vi "Set_Pulse_Manual.vi"() -> ()   [LabVIEW 2021]
uses:
  Drivers/Arduino_Pulse_Generator/Configurate/Channel_Pulse_Stream.ctl
  acefff95-97c1-4a03-be14-0b511ca0e7e1.vi
  db7f351c-eeeb-4ffc-aff2-0ba6d56ef54f.vi
  <vilib>/Comparison/Less/Less Functor/Less Functor.lvclass
panel:
  in  "Filename (.ini)":string="Config_Ver_1\\pulse_sequence.ini"
  out "Initial Array":T1[](array[typedef]) {"channel" min=2 max=13 step=1}
  in  "Reset All":bool
  in  "Reset Channel":bool
  out "Type of channel":string[](array[string])
  out "Times vs channel":dbl[][](array[numeric])
  in  "End configuration":bool
  in  "Stop":dbl
  in  "Start":dbl
  in  "Add Step":bool
  in  "Add Pulse":bool
  in  "Type of channel":u8(ring) items=["probe"=4, "pump"=6, "x pulse"=7]
  # "Note that units of time are not specified there.\nRemember that minimal pulse length is about 3,8 us."
  # "Add pulse with specific type\nbegining (start) and end (stop)"
  # "Add step with specific type\nand time (start)"
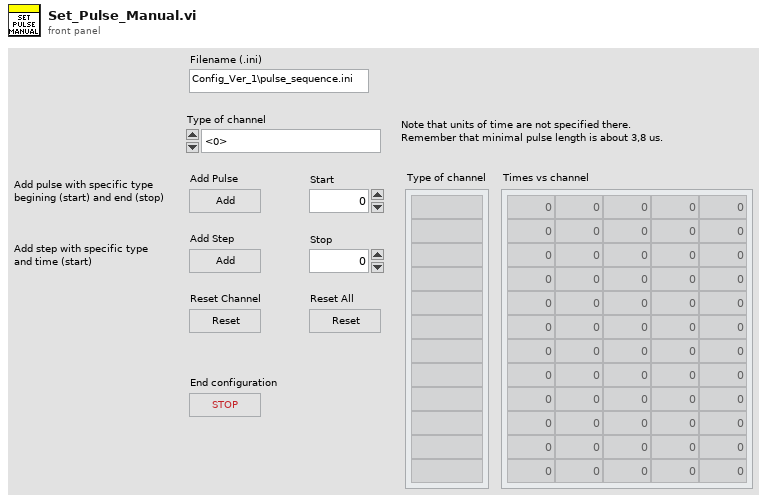
[diagram p1: front panel]
types:
  T1 = typedef "Channel_Pulse_Stream.ctl" = cluster{"Times":dbl[], "channel":u8}
  T2 = typedef "Channels_Map.ctl" = T3[]
  T3 = typedef "Channel_Cluster.ctl" = cluster{"Channel name":string, "Channel":u8}
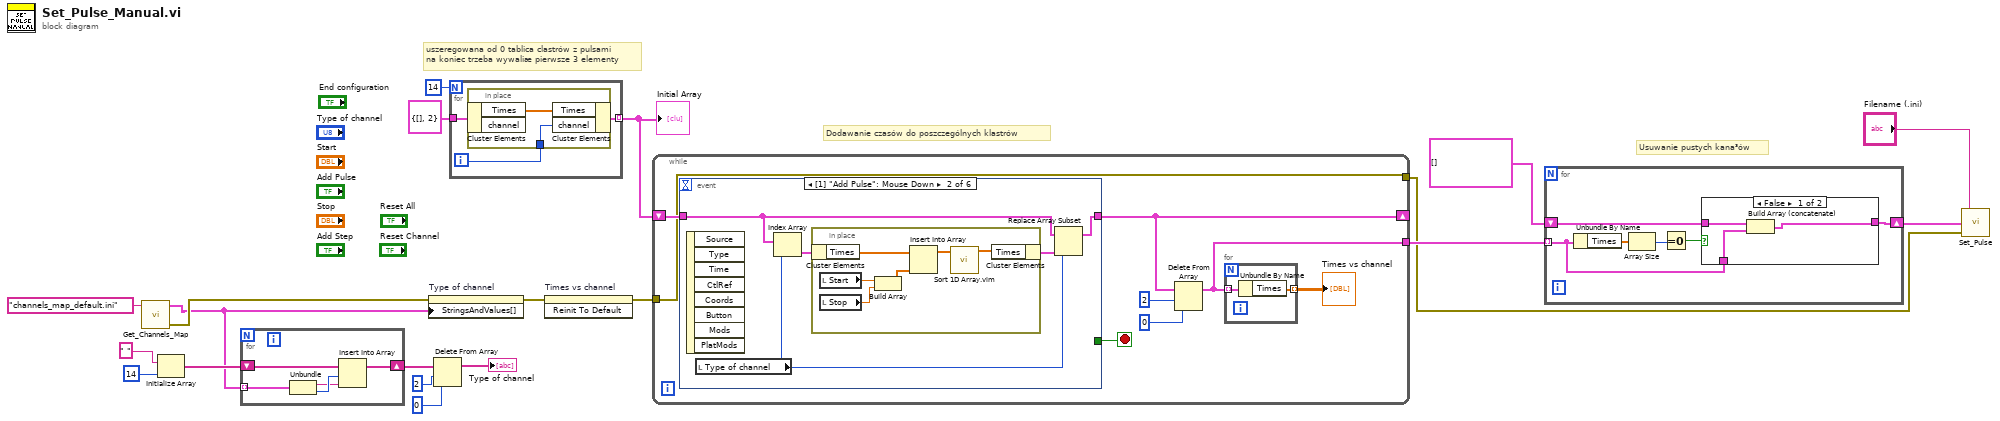
[diagram p0: block diagram]
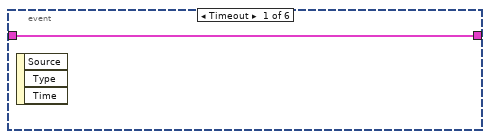
[diagram p3: hidden frame]
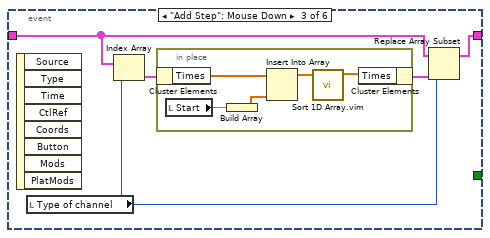
[diagram p4: hidden frame]
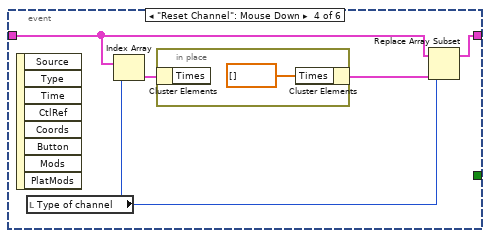
[diagram p5: hidden frame]
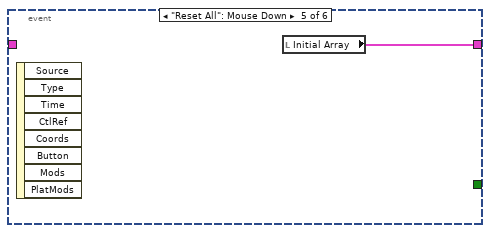
[diagram p6: hidden frame]
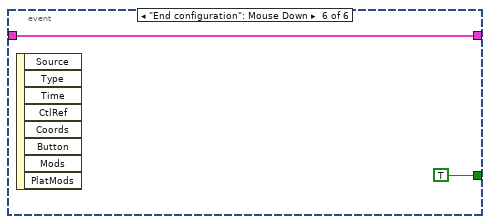
[diagram p7: hidden frame]
diagram:
  # "Usuwanie pustych kana³ów"
  # "uszeregowana od 0 tablica clastrów z pulsami\nna koniec trzeba wywaliæ pierwsze 3 elementy"
  # "Dodawanie czasów do poszczególnych klastrów"
  n1 = call "Get_Channels_Map.vi"("Filename (.ini)"="channels_map_default.ini") -> ("error out"=w6:errorcluster, "Channels Map"=w5:T2)  [unwired: 3 in]
  n2 = Initialize Array(" ", 14 ("dimension size")) -> (w13:string[])
  n3 = for {
    tunnel: w5 -> [w23] mode=indexing
    shift-right: [w22] -> w12
    shift-left: w13 -> [w25]
    n4 = Unbundle(w23) -> ("Channel name"=w21:string, "Channel"=w24:u8)
    n5 = Insert Into Array(array=w25, index=w24, new element=w21) -> (w22:string[])
  }
  n6 = property on="Type of channel" class="Ring (strict)"(error in=w6, "StringsAndValues[]"=w5) -> (error out=w17:errorcluster)  [unwired: 1 in, 1 out]
  n7 = Delete From Array(array=w12, length=2, index=0) -> (array with subset deleted=→"Type of channel":string[])  [unwired: 1 out]
  n8 = for {
    N: 14 -> [_]
    tunnel: T1 {"Times"=[], "channel"=2} ("Channel pulse stream") -> [w28]
    tunnel: [w27] -> w18 mode=indexing
    i -> [w26]
    n9 = in-place {
      in-place-border: w26 -> [w30]
      n10 = in-place-cluster #1(w28) -> ("Times"=w29:dbl[])  [unwired: 1 out]
      n11 = in-place-cluster #1("Times"=w29, "channel"=w30) -> (w27:T1)
    }
  }
  "Initial Array" <- w18
  n12 = invoke on="Times vs channel" class="Arr (strict)" method="Reinit To Default"(error in=w17) -> (error out=w16:errorcluster)  [unwired: 2 in, 2 out]
  n13 = while {
    shift-right: [w34] -> _
    shift-left: w18 -> [w38]
    tunnel: [w32] -> w8
    tunnel: w16 -> [w31]
    tunnel: [w31] -> w2
    stop <- w37 stop-if-true
    n14 = event shown="[1] \"Add Pulse\": Mouse Down" {
      selector: _ -> [_ _ _ _ _ _]
      dyn-events: _ -> [_ _ _ _ _ _]
      timeout: _ -> [_ _ _ _ _ _]
      tunnel: w38 -> [w41 w44 w55 w65 _ w71]
      tunnel: [w41 w42 w53 w63 w69 w71] -> w34
      tunnel: [_ _ _ _ _ TRUE] -> w37
      event Timeout {
        n15 = event-data() -> ()  [unwired: 1 in, 3 out]
      }
      event "Add Pulse": Mouse Down {
        n16 = event-data() -> ()  [unwired: 1 in, 8 out]
        n17 = local read "Type of channel"() -> (w43:u8)
        n18 = Index Array(array=w44, index=w43) -> (element=w46:T1)
        n19 = in-place {
          n20 = in-place-cluster #2(w46) -> ("Times"=w50:dbl[])
          n21 = local read "Start"() -> (w51:dbl)
          n22 = local read "Stop"() -> (w52:dbl)
          n23 = Build Array(w51, w52) -> (w49:dbl[])
          n24 = Insert Into Array(array=w50, new element=w49) -> (w48:dbl[])  [unwired: 1 in]
          n25 = call "Sort 1D Array.vim"("unsorted array"=w48) -> ("sorted array"=w47:dbl[])  [unwired: 10 in]
          n26 = in-place-cluster #2("Times"=w47) -> (w45:T1)
        }
        n27 = Replace Array Subset(array=w44, new element=w45, index=w43) -> (w42:T1[])
      }
      event "Add Step": Mouse Down {
        n28 = event-data() -> ()  [unwired: 1 in, 8 out]
        n29 = local read "Type of channel"() -> (w54:u8)
        n30 = Index Array(array=w55, index=w54) -> (element=w57:T1)
        n31 = in-place {
          n32 = in-place-cluster #3(w57) -> ("Times"=w61:dbl[])
          n33 = local read "Start"() -> (w62:dbl)
          n34 = Build Array(w62) -> (w60:dbl[])
          n35 = Insert Into Array(array=w61, new element=w60) -> (w59:dbl[])  [unwired: 1 in]
          n36 = call "Sort 1D Array.vim"("unsorted array"=w59) -> ("sorted array"=w58:dbl[])  [unwired: 10 in]
          n37 = in-place-cluster #3("Times"=w58) -> (w56:T1)
        }
        n38 = Replace Array Subset(array=w55, new element=w56, index=w54) -> (w53:T1[])
      }
      event "Reset Channel": Mouse Down {
        n39 = event-data() -> ()  [unwired: 1 in, 8 out]
        n40 = local read "Type of channel"() -> (w64:u8)
        n41 = Index Array(array=w65, index=w64) -> (element=w67:T1)
        n42 = in-place {
          n43 = in-place-cluster #4(w67) -> ()  [unwired: 1 out]
          n44 = in-place-cluster #4("Times"=dbl[] []) -> (w66:T1)
        }
        n45 = Replace Array Subset(array=w65, new element=w66, index=w64) -> (w63:T1[])
      }
      event "Reset All": Mouse Down {
        n46 = event-data() -> ()  [unwired: 1 in, 8 out]
        n47 = local read "Initial Array"() -> (w69:T1[])
      }
      event "End configuration": Mouse Down {
        n48 = event-data() -> ()  [unwired: 1 in, 8 out]
      }
    }
    n49 = Delete From Array(array=w34, length=2, index=0) -> (array with subset deleted=w32:T1[])  [unwired: 1 out]
    n50 = for {
      tunnel: w32 -> [w40] mode=indexing
      tunnel: [w39] -> w33 mode=indexing
      n51 = Unbundle By Name(w40) -> ("Times"=w39:dbl[])
    }
    "Times vs channel" <- w33
  }
  n52 = for {
    shift-right: [w74] -> w4
    shift-left: T1[] [] -> [w73]
    tunnel: w8 -> [w72] mode=indexing
    n53 = Unbundle By Name(w72) -> ("Times"=w77:dbl[])
    n54 = Array Size(array=w77) -> (size(s)=w76:i32)
    n55 = Equal To 0?(x=w76) -> (x = 0?=w75:bool)
    n56 = case shown="False" w75 {
      tunnel: w73 -> [w80 w81]
      tunnel: [w78 w81] -> w74
      tunnel: w72 -> [w79 _]
      frame False {
        n57 = Build Array (concatenate)(w80, w79) -> (w78:T1[])
      }
      frame True {
      }
    }
  }
  n58 = call "Set_Pulse.vi"("error in"=w2, "Pulse sequence"=w4, "Filename (.ini)"="Filename (.ini)") -> ()  [unwired: 1 in, 1 out]
